vi "FGV.vi"(7 "Action":enum16{"Initialize", "Read", "Write"}(ring), 8 "error in (no error)":errorcluster, 9 "Successful":bool, 11 "Read Data":string) -> (0 "error out":errorcluster, 1 "Successful":bool, 3 "Read Data":string)   [LabVIEW 2025, in "Interface Functions.lvlib"]
uses:
  Interface Functions.lvlib
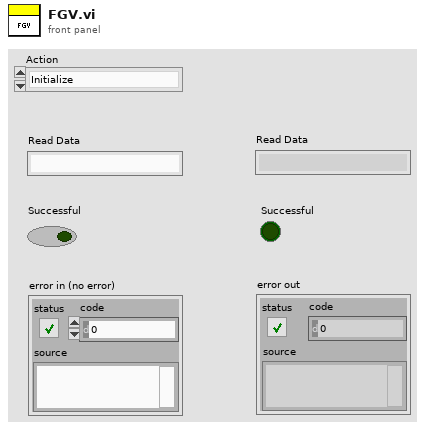
[diagram p1: front panel]
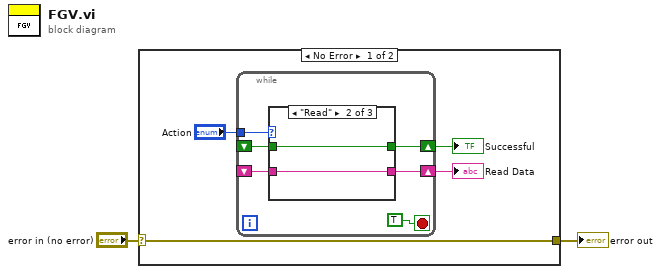
[diagram p0: block diagram]
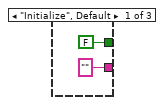
[diagram p2: hidden frame]
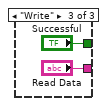
[diagram p3: hidden frame]
diagram:
  n1 = case shown="No Error" "error in (no error)" {
    selector: "error in (no error)" -> [w5 w19]
    tunnel: [w5 w19] -> w1
    frame No Error {
      n2 = while {
        shift-right: [w10] -> w4
        shift-left: _ -> [w11]
        tunnel: "Action" -> [w12]
        shift-right: [w8] -> w3
        shift-left: _ -> [w7]
        stop <- TRUE stop-if-true
        n3 = case shown="\"Read\"" w12 {
          tunnel: w11 -> [_ w16 _]
          tunnel: ["" ("Read Data") w16 "Read Data"] -> w10
          tunnel: [FALSE ("Successful") w15 "Successful"] -> w8
          tunnel: w7 -> [_ w15 _]
          frame "Initialize", Default {
          }
          frame "Read" {
          }
          frame "Write" {
          }
        }
      }
      "Read Data" <- w4
      "Successful" <- w3
    }
    frame Error {
    }
  }
  "error out" <- w1
